vi "AI Initialize.vi"(8 "error in (no error)":errorcluster, 10 "Custom XML":string, 11 "Device Ref in":T1 format="%.0x") -> (0 "error out":errorcluster, 3 "Device Ref out":T1 format="%.0x")   [LabVIEW 2013]
uses:
  <vilib>/K2Labs/HiLab API/Custom Device API/Controls/Custom Device Item Reference.ctl
  <vilib>/K2Labs/HiLab API/Custom Device API/Configuration/Item Properties/Set Item Property/Set Item Property.xnode
  <vilib>/K2Labs/HiLab API/Custom Device API/Custom Device API Library.lvlib
  <vilib>/K2Labs/HiLab API/Custom Device API/Controls/Custom Device Channel Dimensions.ctl
  <vilib>/K2Labs/HiLab API/Custom Device API/Controls/Custom Device Channel Type.ctl
  <vilib>/K2Labs/HiLab API/Custom Device API/Controls/Custom Device Channel.ctl
  <vilib>/K2Labs/HiLab API/Custom Device API/Configuration/Item Properties/Set Item Property/Set Item Property(String).vi
  <vilib>/K2Labs/HiLab API/Custom Device API/Configuration/Item Properties/Set Item Property/Set Item Property(DependentNode).vi
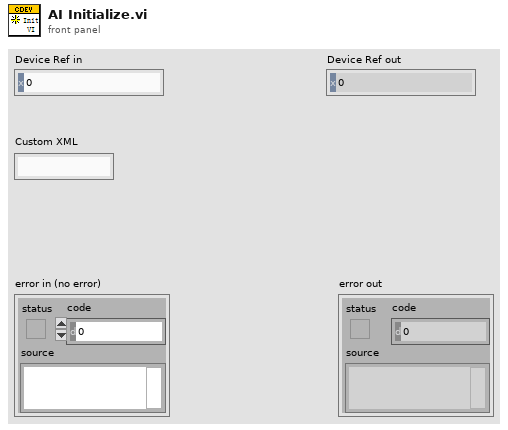
[diagram p1: front panel]
types:
  T1 = typedef "Custom Device API Library.lvlib/Custom Device Item Reference.ctl" = u64
  T2 = typedef "Custom Device API Library.lvlib/Custom Device Channel.ctl" = cluster{"DefaultValue":dbl[], "Dimensions":T3, "Units":string, "Type":T4}
  T3 = typedef "Custom Device API Library.lvlib/Custom Device Channel Dimensions.ctl" = cluster{"Row":i32, "Column":i32}
  T4 = typedef "Custom Device API Library.lvlib/Custom Device Channel Type.ctl" = enum16{"Input", "Output"}
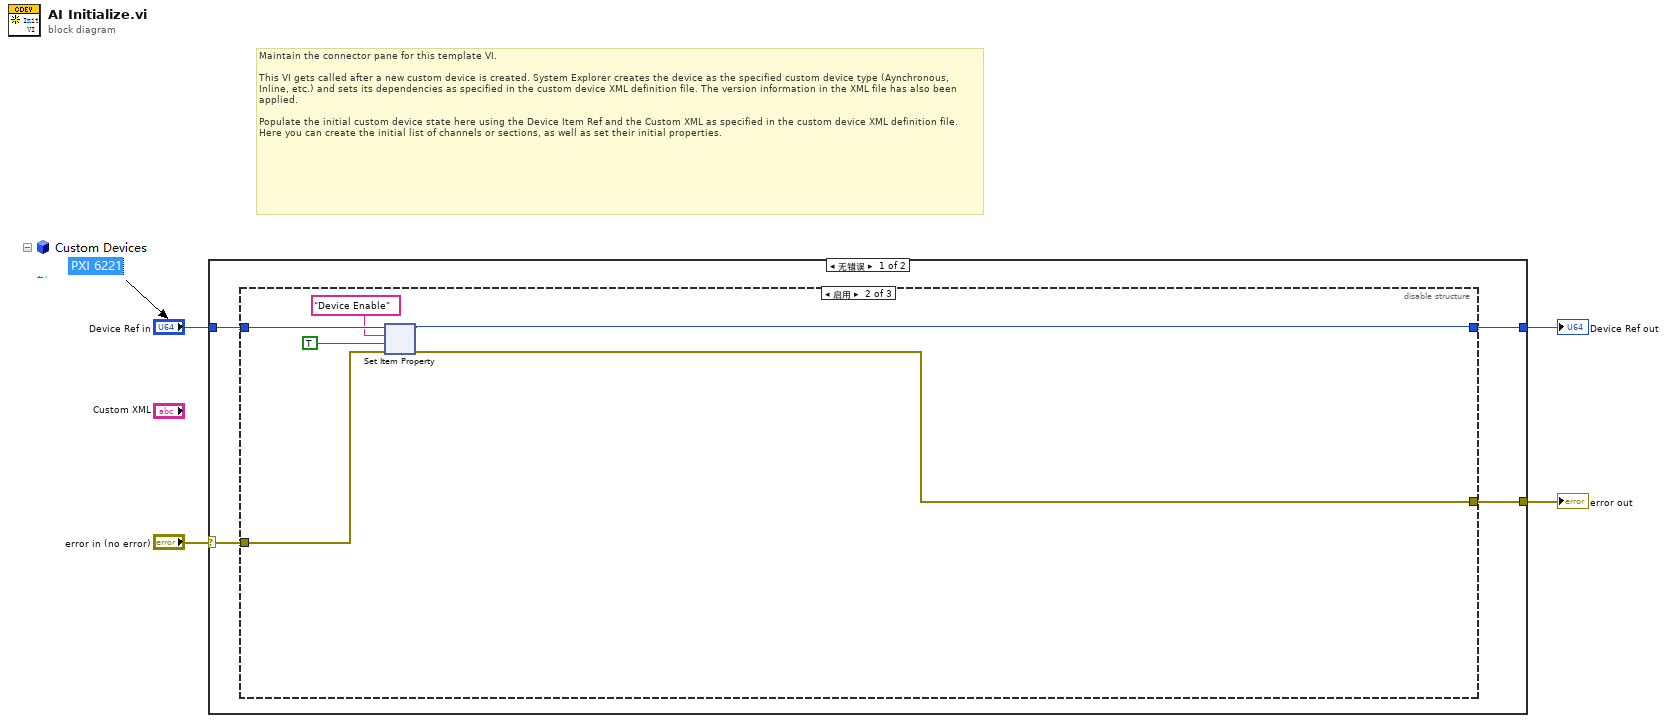
[diagram p0: block diagram]
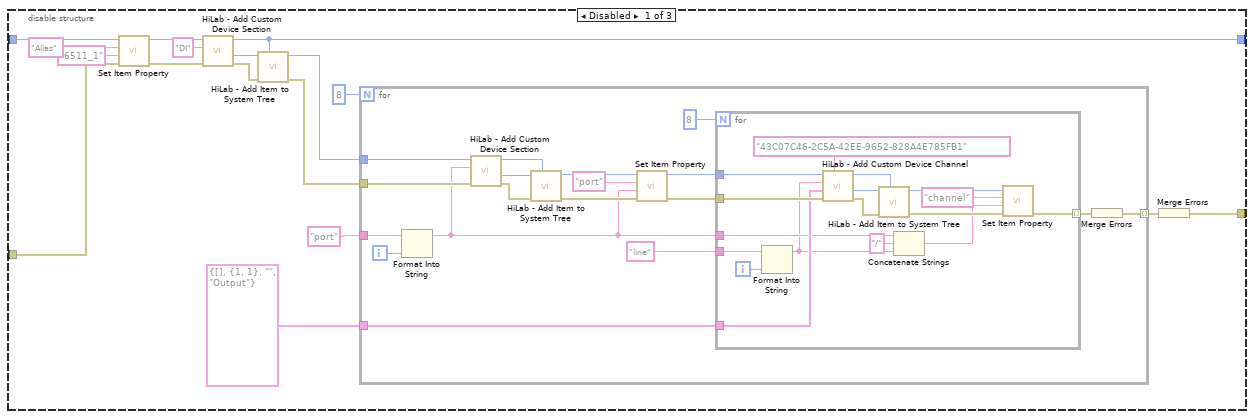
[diagram p2: hidden frame]
diagram:
  # "Maintain the connector pane for this template VI.\n\nThis VI gets called after a new custom device is created. System Explorer creates the device as the specified custom device type (Aynchronous, Inline, etc.) and sets its dependencies as specified in the custom device XML definition file. The version information in the XML file has also been applied.\n\nPopulate the initial custom device state here using the Device Item Ref and the Custom XML as specified in the custom device XML definition file. Here you can create the initial list of channels or sections, as well as set their initial properties."
  n1 = case shown="无错误" "error in (no error)" {
    selector: "error in (no error)" -> [w5 w96]
    tunnel: [w8 w96] -> w3
    tunnel: "Device Ref in" -> [w6 w95]
    tunnel: [w7 w95] -> w1
    frame No Error {
      n2 = disable-structure shown="启用" {
        disable-tunnel: [w14 w61 _] -> w8
        disable-tunnel: [w12 w62 _] -> w7
        disable-tunnel: w6 -> [w11 w66 _]
        disable-tunnel: w5 -> [w10 w65 _]
        frame Disabled {
          n3 = call-poly <vilib>:"Set Item Property.vi"("error in (no error)"=w10, "Value"="6511_1", "Property Name"="Alias", "Item Ref in"=w11) -> ("error out"=w16:errorcluster, "Item Ref out"=w13:T1)  [unwired: 5 in, 1 out]
          n4 = call <vilib>:"HiLab - Add Custom Device Section.vi"("error in (no error)"=w16, "Section Name"="DI", "Parent Ref in"=w13) -> ("error out"=w23:errorcluster, "Channel Ref"=w24:T1, "Parent Ref out"=w12:T1)  [unwired: 5 in, 1 out]
          n5 = call <vilib>:"HiLab - Add Item to System Tree.vi"("Parent Item Ref"=w12, "error in (no error)"=w23, "Item Ref in"=w24) -> ("error out"=w21:errorcluster, "Item Ref out"=w22:T1)  [unwired: 7 in]
          n6 = for {
            N: 8 -> [_]
            tunnel: w22 -> [w32]
            tunnel: w21 -> [w31]
            tunnel: "port" ("Section Name") -> [w40]
            tunnel: T2 {"DefaultValue"=[], "Dimensions"={"Row"=1, "Column"=1}, "Units"="", "Type"=enum."Output"} ("Channel") -> [w39]
            tunnel: [w42] -> w15 mode=indexing
            i -> [w41]
            n7 = Format Into String(initial string=w40, w41) -> (resulting string=w27:string)  [unwired: 2 in, 1 out]
            n8 = call <vilib>:"HiLab - Add Custom Device Section.vi"("error in (no error)"=w31, "Section Name"=w27, "Parent Ref in"=w32) -> ("error out"=w28:errorcluster, "Channel Ref"=w29:T1, "Parent Ref out"=w30:T1)  [unwired: 5 in, 1 out]
            n9 = call <vilib>:"HiLab - Add Item to System Tree.vi"("Parent Item Ref"=w30, "error in (no error)"=w28, "Item Ref in"=w29) -> ("error out"=w36:errorcluster, "Item Ref out"=w37:T1)  [unwired: 7 in]
            n10 = call-poly <vilib>:"Set Item Property.vi"("error in (no error)"=w36, "Value"=w27, "Property Name"="port", "Item Ref in"=w37) -> ("error out"=w35:errorcluster, "Item Ref out"=w33:T1)  [unwired: 5 in, 1 out]
            n11 = for {
              N: 8 -> [_]
              tunnel: w33 -> [w60]
              tunnel: w35 -> [w59]
              tunnel: w39 -> [w55]
              tunnel: [w50] -> w43 mode=indexing
              tunnel: w27 -> [w47]
              tunnel: "line" ("字符串") -> [w48]
              i -> [w49]
              n12 = Format Into String(initial string=w48, w49) -> (resulting string=w46:string)  [unwired: 2 in, 1 out]
              n13 = call <vilib>:"HiLab - Add Custom Device Channel.vi"("GUID (Default Channel)"="43C07C46-2C5A-42EE-9652-828A4E785FB1", "error in (no error)"=w59, "Channel"=w55, "Channel Name"=w46, "Parent Ref in"=w60) -> ("error out"=w56:errorcluster, "Channel Ref"=w58:T1, "Parent Ref out"=w57:T1)  [unwired: 3 in, 1 out]
              n14 = call <vilib>:"HiLab - Add Item to System Tree.vi"("Parent Item Ref"=w57, "error in (no error)"=w56, "Item Ref in"=w58) -> ("error out"=w53:errorcluster, "Item Ref out"=w54:T1)  [unwired: 7 in]
              n15 = Concatenate Strings(w47, "/" ("字符串"), w46) -> (w45:string)
              n16 = call-poly <vilib>:"Set Item Property.vi"("error in (no error)"=w53, "DependentNode Path"=w45, "Property Name"="channel", "Item Ref in"=w54) -> ("error out"=w50:errorcluster)  [unwired: 5 in, 2 out]
            }
            n17 = Merge Errors(w43) -> (w42:errorcluster)
          }
          n18 = Merge Errors(w15) -> (w14:errorcluster)
        }
        frame Enabled {
          n19 = xnode "Set Item Property"("Item Ref in"=w66, "error in (no error)"=w65, "Property Name"="Device Enable", "Value"=TRUE) -> ("Item Ref out"=w62:T1, "error out"=w61:errorcluster)  [unwired: 1 out]
        }
        frame Disabled {
        }
      }
    }
    frame Error {
    }
  }
  "Device Ref out" <- w1
  "error out" <- w3
